vi "TDT-Enumerate Device Names.vi"(11 "error in (no error)":errorcluster, 13 "Acceptable Devices":T1[](array[typedef])=[enum."RX6", enum."RZ5", enum."RZ6"]) -> (8 "Device names":string[](array[string]), 15 "error out":errorcluster)   [LabVIEW 2020]
uses:
  Typedefs/TDT-Device ID.ctl
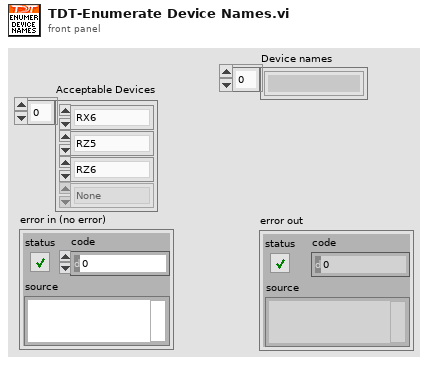
[diagram p1: front panel]
types:
  T1 = typedef "TDT-Device ID.ctl" = enum16{"None", "PA5", "RP2", "RL2", "RA16", "RV8", "RX5", "RX6", "RX7", "RX8", "RZ2", "RZ5", "RZ6"}
  T2 = typedef "TDT-Output source.ctl" = cluster{"Device":T1, "Num":i32}
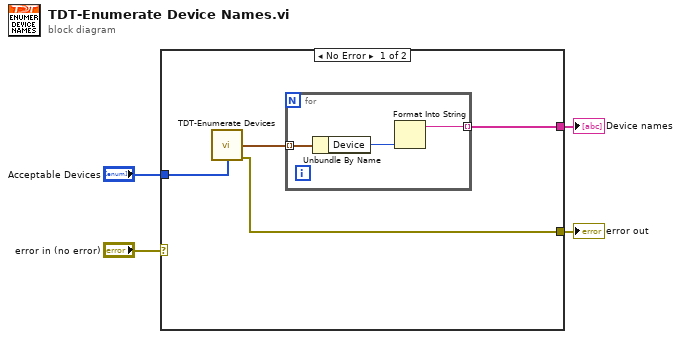
[diagram p0: block diagram]
diagram:
  n1 = case shown="No Error" "error in (no error)" {
    selector: "error in (no error)" -> [_ w12]
    tunnel: "Acceptable Devices" -> [w8 _]
    tunnel: [w7 w12] -> w2
    tunnel: [w5 _] -> w1
    frame No Error {
      n2 = call "TDT-Enumerate Devices.vi"("Acceptable Devices"=w8) -> ("Devices"=w6:T2[], "error out"=w7:errorcluster)  [unwired: 13 in]
      n3 = for {
        tunnel: w6 -> [w11] mode=indexing
        tunnel: [w9] -> w5 mode=indexing
        n4 = Unbundle By Name(w11) -> ("Device"=w10:T1)
        n5 = Format Into String(w10) -> (resulting string=w9:string)  [unwired: 3 in, 1 out]
      }
    }
    frame Error {
    }
  }
  "error out" <- w2
  "Device names" <- w1
